vi "MB Ethernet Wait on Query.vi"(10 "Timeout":i32=5000, 11 "Connection ID":refnum<k5>) -> ()   [LabVIEW 2010]
uses:
  NI_Modbus.llb/MB RefCount Function.ctl
  NI_Modbus.llb/MB Ethernet Connection Function.ctl
panel:
  # "VI Name: MB Ethernet Wait on Query.vi\nPurpose: Serves a Modbus TCP query.\nReentrant VI called dynamically, so that multiple\nqueries can be served in parallel."
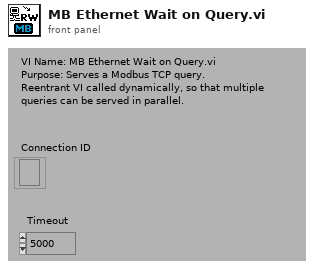
[diagram p1: front panel]
types:
  T1 = typedef "MB RefCount Function.ctl" = enum16{"Init", "Add", "Remove", "Is Running?"}
  T2 = typedef "MB Ethernet Connection Function.ctl" = enum16{"Init", "Add Connection", "Get All Connections", "Delete Connection"}
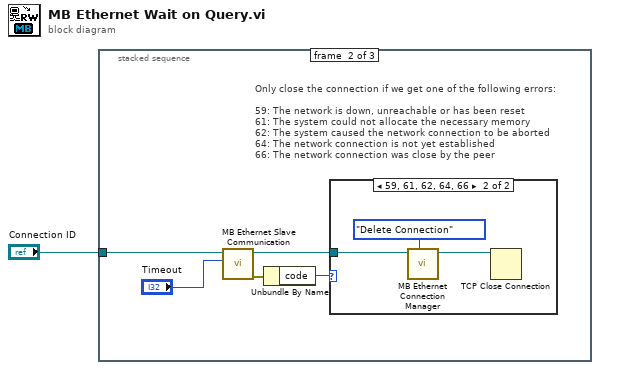
[diagram p0: block diagram]
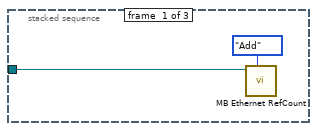
[diagram p2: hidden frame]
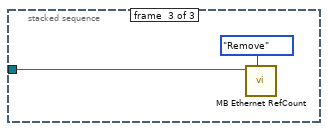
[diagram p4: hidden frame]
diagram:
  n1 = stacked-sequence {
    tunnel: "Connection ID" -> [w2 w6 w12]
    frame #0 {
      n2 = call "MB Ethernet RefCount.vi"("Function"=MB_RefCount_Function."Add", "Connection ID"=w2) -> ()  [unwired: 10 out]
    }
    frame #1 {
      # "Only close the connection if we get one of the following errors:\n\n59: The network is down, unreachable or has been reset\n61: The system could not allocate the necessary memory\n62: The system caused the network connection to be aborted\n64: The network connection is not yet established\n66: The network connection was close by the peer"
      n3 = call "MB Ethernet Slave Communication.vi"("Timeout"="Timeout", "Connection ID"=w6) -> ("error out"=w5:errorcluster, "Connection ID (dup)"=w8:refnum<k5>)  [unwired: 1 in, 7 out]
      n4 = Unbundle By Name(w5) -> ("code"=w4:i32)
      n5 = case shown="59, 61, 62, 64, 66" w4 {
        tunnel: w8 -> [_ w10]
        frame 0, Default {
        }
        frame 59, 61, 62, 64, 66 {
          n6 = call "MB Ethernet Connection Manager.vi"("Function"=MB_Ethernet_Connection_Function."Delete Connection", "Connection ID"=w10) -> ("Connection ID to Delete"=w9:refnum<k5>)  [unwired: 1 in, 8 out]
          n7 = TCP Close Connection(connection ID=w9) -> ()  [unwired: 1 in, 3 out]
        }
      }
    }
    frame #2 {
      n8 = call "MB Ethernet RefCount.vi"("Function"=MB_RefCount_Function."Remove", "Connection ID"=w12) -> ()  [unwired: 10 out]
    }
  }
